vi "Get Hi Low Time By ID V.vi"(8 "error in (no error)":errorcluster, 10 "dateTimeValue":T1, 11 "weatherDataID":u32) -> (0 "error out":errorcluster, 2 "dateTimeValue out":T1, 3 "function return":i16)   [LabVIEW 2009, in "VantagePro.lvlib"]
doc: "DllAccess short int _stdcall GetHiLowTimeByID_V(DWORD weatherDataID, DateTimeStamp *dateTimeValue);"
uses:
  VantagePro.lvlib
  <userlib>/VantagePro/VantagePro.dll
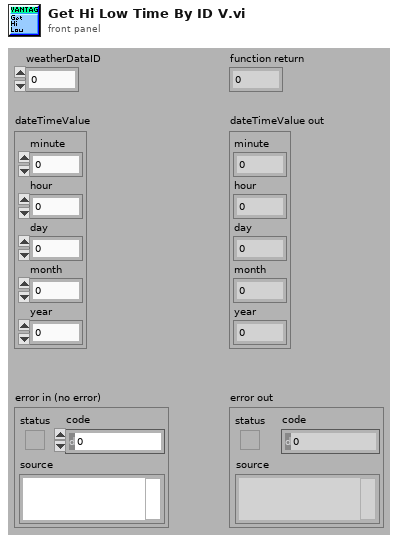
[diagram p1: front panel]
types:
  T1 = cluster{"minute":i32, "hour":i32, "day":i32, "month":i32, "year":i32}
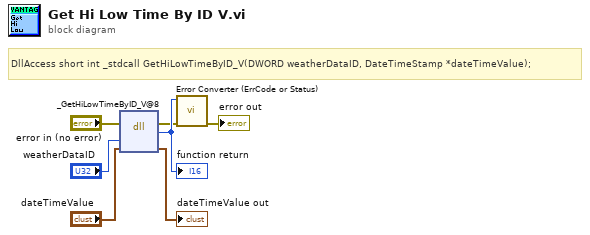
[diagram p0: block diagram]
diagram:
  # "DllAccess short int _stdcall GetHiLowTimeByID_V(DWORD weatherDataID, DateTimeStamp *dateTimeValue);"
  n1 = dll-call lib="C:/Program Files/National Instruments/LabVIEW 2010/user.lib/VantagePro/VantagePro.*" fn="_GetHiLowTimeByID_V@8"(error in="error in (no error)", "weatherDataID"="weatherDataID", "dateTimeValue"="dateTimeValue") -> (error out=w2:errorcluster, w7:i16, "dateTimeValue"=→"dateTimeValue out":T1)  [unwired: 3 in, 1 out]
  "function return" <- w7
  n2 = call "Error Converter (ErrCode or Status).vi"("error in (no error)"=w2, "error code"=w7) -> ("error out"=→"error out":errorcluster)  [unwired: 9 in]
